vi "LH6HD_inycom.vi"(6 "DeviceAddress":u8, 8 "error in (no error)":errorcluster, 9 "Reader Port":u16, 10 "IP Address":string, 11 "Action":enum16{"Init", "Start", "Read", "Stop", "Exit"}(ring)) -> (0 "error out":errorcluster, 3 "Tag":string)   [LabVIEW 2015]
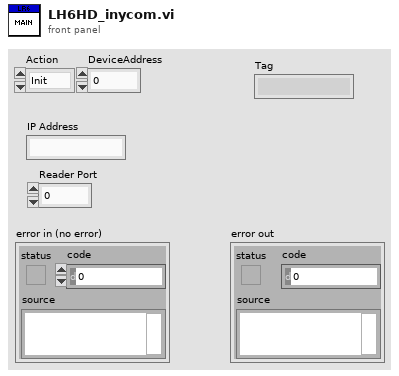
[diagram p1: front panel]
types:
  T1 = enum16{"IniciarLectura", "SolicitarEstado", "SolicitarTag", "Inhibir"}
  T2 = enum16{"Unknown", "Estado OK", "Ocupado", "Inhibit OK", "Waiting", "Reset"}
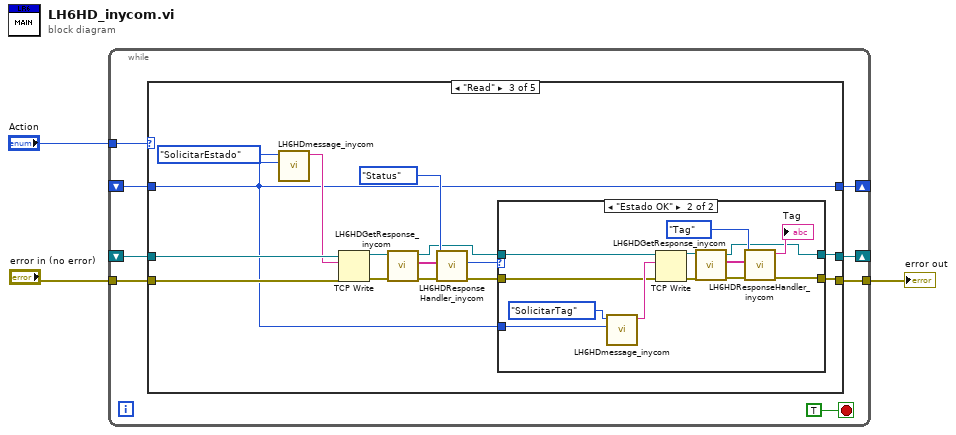
[diagram p0: block diagram]
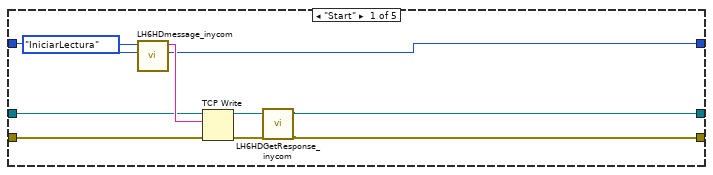
[diagram p2: hidden frame]
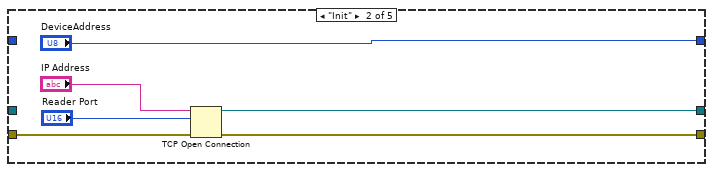
[diagram p3: hidden frame]
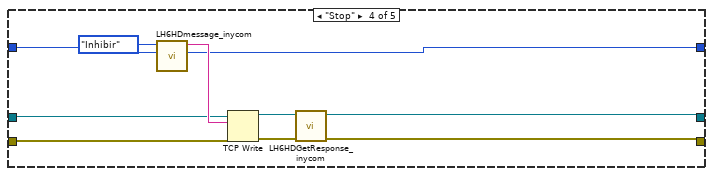
[diagram p5: hidden frame]
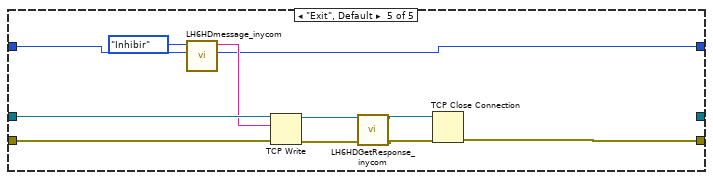
[diagram p6: hidden frame]
diagram:
  n1 = while {
    tunnel: "Action" -> [w10]
    tunnel: "error in (no error)" -> [w9]
    tunnel: [w8] -> w1
    shift-right: [w7] -> _
    shift-left: _ -> [w6]
    shift-right: [w5] -> _
    shift-left: _ -> [w4]
    stop <- TRUE stop-if-true
    n2 = case shown="\"Read\"" w10 {
      tunnel: w9 -> [w19 w24 w41 w63 w75]
      tunnel: [w13 w23 w29 w58 w74] -> w8
      tunnel: [w12 w22 w28 w57 _] -> w7
      tunnel: w6 -> [w17 _ w40 w62 w73]
      tunnel: [w16 "DeviceAddress" w30 w61 w70] -> w5
      tunnel: w4 -> [w16 _ w30 w61 w70]
      frame "Start" {
        n3 = call "LH6HDmessage_inycom.vi"("DeviceAddress"=w16, "MessageType"=T1."IniciarLectura") -> ("Message"=w18:string)  [unwired: 9 in]
        n4 = TCP Write(connection ID=w17, data in=w18, error in (no error)=w19) -> (connection ID out=w14:refnum<k5>, error out=w15:errorcluster)  [unwired: 1 in, 1 out]
        n5 = call "LH6HDGetResponse_inycom.vi"("error in (no error)"=w15, "TCP Network Connection in"=w14) -> ("error out"=w13:errorcluster, "TCP Network Connection out"=w12:refnum<k5>)  [unwired: 7 in, 1 out]
      }
      frame "Init" {
        n6 = TCP Open Connection(address="IP Address", remote port or service name="Reader Port", error in (no error)=w24) -> (connection ID=w22:refnum<k5>, error out=w23:errorcluster)  [unwired: 2 in]
      }
      frame "Read" {
        n7 = call "LH6HDmessage_inycom.vi"("DeviceAddress"=w30, "MessageType"=T1."SolicitarEstado") -> ("Message"=w38:string)  [unwired: 9 in]
        n8 = TCP Write(connection ID=w40, data in=w38, error in (no error)=w41) -> (connection ID out=w36:refnum<k5>, error out=w37:errorcluster)  [unwired: 1 in, 1 out]
        n9 = call "LH6HDGetResponse_inycom.vi"("error in (no error)"=w37, "TCP Network Connection in"=w36) -> ("error out"=w34:errorcluster, "Response"=w35:string[], "TCP Network Connection out"=w27:refnum<k5>)  [unwired: 7 in]
        n10 = call "LH6HDResponseHandler_inycom.vi"("error in (no error)"=w34, "Response"=w35, "Enum in"=enum16{"Tag", "Status"}."Status") -> ("error out"=w31:errorcluster, "Enum out"=w32:T2)  [unwired: 6 in, 1 out]
        n11 = case shown="\"Estado OK\"" w32 {
          tunnel: w31 -> [w43 w53]
          tunnel: w27 -> [w42 w52]
          tunnel: w30 -> [_ w56]
          tunnel: [w43 w46] -> w29
          tunnel: [w42 w44] -> w28
          frame "Unknown", Default {
          }
          frame "Estado OK" {
            n12 = call "LH6HDmessage_inycom.vi"("DeviceAddress"=w56, "MessageType"=T1."SolicitarTag") -> ("Message"=w54:string)  [unwired: 9 in]
            n13 = TCP Write(connection ID=w52, data in=w54, error in (no error)=w53) -> (connection ID out=w48:refnum<k5>, error out=w49:errorcluster)  [unwired: 1 in, 1 out]
            n14 = call "LH6HDGetResponse_inycom.vi"("error in (no error)"=w49, "TCP Network Connection in"=w48) -> ("error out"=w51:errorcluster, "Response"=w50:string[], "TCP Network Connection out"=w44:refnum<k5>)  [unwired: 7 in]
            n15 = call "LH6HDResponseHandler_inycom.vi"("error in (no error)"=w51, "Response"=w50, "Enum in"=enum16{"Tag", "Status"}."Tag") -> ("error out"=w46:errorcluster, "String"=→"Tag":string)  [unwired: 6 in, 1 out]
          }
        }
      }
      frame "Stop" {
        n16 = call "LH6HDmessage_inycom.vi"("DeviceAddress"=w61, "MessageType"=T1."Inhibir") -> ("Message"=w64:string)  [unwired: 9 in]
        n17 = TCP Write(connection ID=w62, data in=w64, error in (no error)=w63) -> (connection ID out=w60:refnum<k5>, error out=w59:errorcluster)  [unwired: 1 in, 1 out]
        n18 = call "LH6HDGetResponse_inycom.vi"("error in (no error)"=w59, "TCP Network Connection in"=w60) -> ("error out"=w58:errorcluster, "TCP Network Connection out"=w57:refnum<k5>)  [unwired: 7 in, 1 out]
      }
      frame "Exit", Default {
        n19 = call "LH6HDmessage_inycom.vi"("DeviceAddress"=w70, "MessageType"=T1."Inhibir") -> ("Message"=w71:string)  [unwired: 9 in]
        n20 = TCP Write(connection ID=w73, data in=w71, error in (no error)=w75) -> (connection ID out=w67:refnum<k5>, error out=w69:errorcluster)  [unwired: 1 in, 1 out]
        n21 = call "LH6HDGetResponse_inycom.vi"("error in (no error)"=w69, "TCP Network Connection in"=w67) -> ("error out"=w68:errorcluster, "TCP Network Connection out"=w66:refnum<k5>)  [unwired: 7 in, 1 out]
        n22 = TCP Close Connection(connection ID=w66, error in (no error)=w68) -> (error out=w74:errorcluster)  [unwired: 1 in, 1 out]
      }
    }
  }
  "error out" <- w1
